vi "AssertConnectorPanesMatchTemplateFiles.vi"(6 "terminal subset acceptable (false)":bool, 8 "error in (no error)":errorcluster, 9 "absolute custom device xml file":path, 10 "Array":T1(array[cluster]), 11 "TestCase in":refnum<class "TestCase.lvclass">) -> (0 "error out":errorcluster, 3 "TestCase out":refnum<class "TestCase.lvclass">)   [LabVIEW 2016, in "VeriStandTestUtilities.lvlib"]
uses:
  VeriStandTestUtilities.lvlib
  <vilib>/addons/_JKI Toolkits/VI Tester/TestCase.llb/TestCase.lvclass
  <userlib>/_OpenG.lib/array/array.llb/Remove Duplicates from 1D Array (Variant)__ogtk.vi
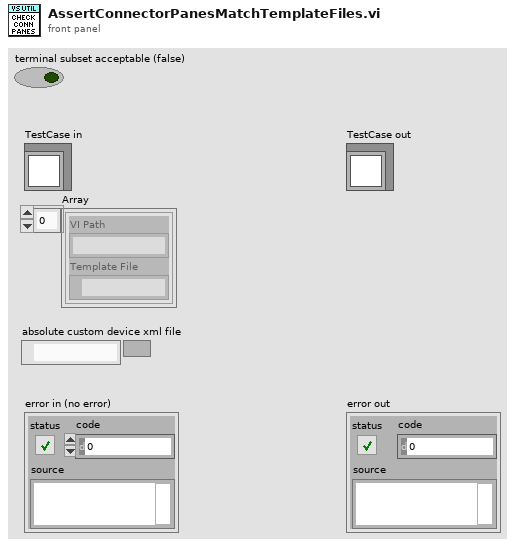
[diagram p1: front panel]
types:
  T1 = cluster{"VI Path":string, "Template File":path}[]
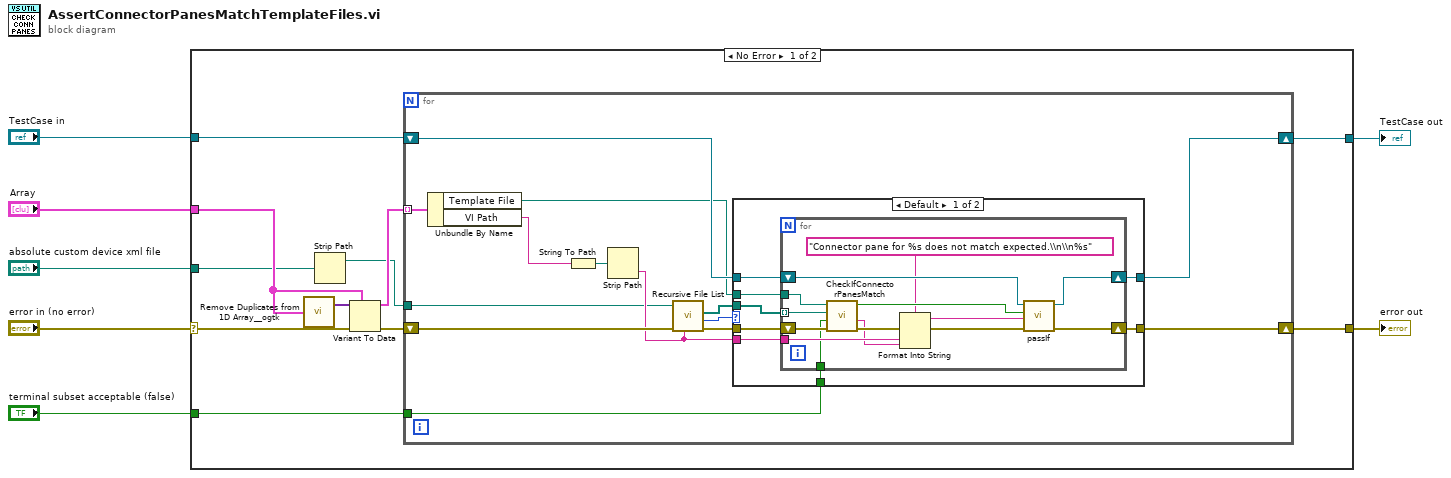
[diagram p0: block diagram]
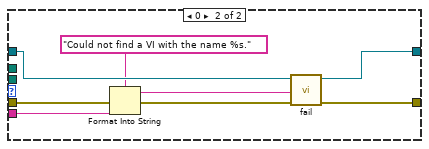
[diagram p2: hidden frame]
diagram:
  n1 = case shown="No Error" "error in (no error)" {
    selector: "error in (no error)" -> [w11 w64]
    tunnel: "absolute custom device xml file" -> [w9 _]
    tunnel: [w18 w63] -> w6
    tunnel: "TestCase in" -> [w17 w63]
    tunnel: [w12 w64] -> w4
    tunnel: "Array" -> [w14 _]
    tunnel: "terminal subset acceptable (false)" -> [w16 _]
    frame No Error {
      n2 = call-poly <userlib>:"Remove Duplicates from 1D Array__ogtk.vi"("Input Array"=w14) -> ("Output Array"=w15:variant[])  [unwired: 1 out]
      n3 = Strip Path(path=w9) -> (stripped path=w8:path)  [unwired: 1 out]
      n4 = Variant To Data(error in=w11, type=w14, Variant=w15) -> (data=w13:T1, error out=w10:errorcluster)
      n5 = for {
        shift-right: [w30] -> w12
        shift-left: w10 -> [w25]
        tunnel: w13 -> [w29] mode=indexing
        shift-right: [w32] -> w18
        shift-left: w17 -> [w31]
        tunnel: w16 -> [w28]
        tunnel: w8 -> [w23]
        n6 = Unbundle By Name(w29) -> ("Template File"=w19:path, "VI Path"=w26:string)
        n7 = String To Path(string=w26) -> (path=w27:path)
        n8 = Strip Path(path=w27) -> (name=w24:string)  [unwired: 1 out]
        n9 = call <vilib>:"Recursive File List.vi"("pattern"=w24, "error in (no error)"=w25, "Folder Path"=w23) -> ("error out"=w21:errorcluster, "Number of Files"=w22:i32, "All Files in Dir"=w20:path[])  [unwired: 4 in, 2 out]
        n10 = case shown="Default" w22 {
          tunnel: w21 -> [w40 w58]
          tunnel: [w38 w62] -> w30
          tunnel: w20 -> [w35 _]
          tunnel: w19 -> [w39 _]
          tunnel: w31 -> [w37 w61]
          tunnel: [w36 w60] -> w32
          tunnel: w24 -> [w34 w59]
          tunnel: w28 -> [w33 _]
          frame Default {
            n11 = for {
              tunnel: w39 -> [w53]
              shift-right: [w51] -> w38
              shift-left: w40 -> [w54]
              shift-right: [w49] -> w36
              shift-left: w37 -> [w50]
              tunnel: w35 -> [w48] mode=indexing
              tunnel: w34 -> [w46]
              tunnel: w33 -> [w41]
              n12 = call "CheckIfConnectorPanesMatch.vi"("error in (no error)"=w54, "terminal subset acceptable (false)"=w41, "actual connector pane vi"=w48, "expected connector pane vi"=w53) -> ("error out"=w44:errorcluster, "mismatch explanation"=w42:string, "connector panes match"=w52:bool)  [unwired: 5 in]
              n13 = Format Into String(format string="Connector pane for %s does not match expected.\\n\\n%s" ("connector pane mismatch error"), error in=w44, w46, w42) -> (resulting string=w45:string, error out=w47:errorcluster)  [unwired: 1 in]
              n14 = call-dynamic "passIf.vi"("error in (no error)"=w47, "message (\"\")"=w45, "pass"=w52, "TestCase in"=w50) -> ("error out"=w51:errorcluster, "TestCase out"=w49:refnum<class "TestCase.lvclass">)  [unwired: 6 in]
            }
          }
          frame 0 {
            n15 = Format Into String(format string="Could not find a VI with the name %s." ("no matches error"), error in=w58, w59) -> (resulting string=w56:string, error out=w57:errorcluster)  [unwired: 1 in]
            n16 = call-dynamic "fail.vi"("error in (no error)"=w57, "message (\"\")"=w56, "TestCase in"=w61) -> ("error out"=w62:errorcluster, "TestCase out"=w60:refnum<class "TestCase.lvclass">)  [unwired: 7 in]
          }
        }
      }
    }
    frame Error {
    }
  }
  "TestCase out" <- w6
  "error out" <- w4
